vi "GetRoom.vi"(7 "Room Commands":T1, 8 "error in (no error)":errorcluster, 11 "Room Number":i32) -> (0 "error out":errorcluster, 2 "Flags JSON":string)   [LabVIEW 2015, in "RestApi.lvlib"]
uses:
  RestApi.lvlib
  TypeDef/GetRoomCommands.ctl
  TypeDef/FGVAction.ctl
  <vilib>/httpClient/LabVIEWHTTPClient.lvlib
panel:
  out "URL":string
  out "headers":string
  # "http://127.0.0.1:8001/WebService1/ReadFlag?Room={value}"
  # "http://127.0.0.1:8001/RivERWebService/"
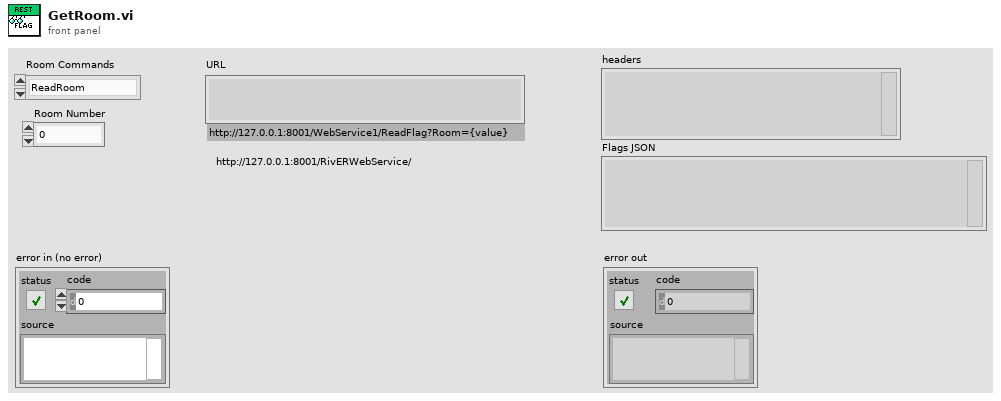
[diagram p1: front panel]
types:
  T1 = typedef "RestApi.lvlib/GetRoomCommands.ctl" = enum16{"ReadRoom", "ReadFlag", "ReadFlagState", "ReadFlagColor", "ReadBedVacant", "ReadPersonnel", "ReadRequests", "ReadBeaconID", "ReadBedURL"}
  T2 = typedef "FGVAction.ctl" = enum16{"Get", "Set"}
  T3 = typedef "LabVIEWHTTPClient.lvlib/ClientHandle.ctl" = refnum<k1>
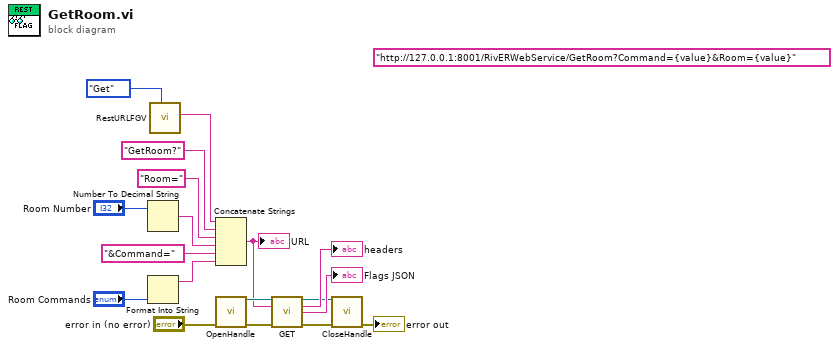
[diagram p0: block diagram]
diagram:
  (unwired) "http://127.0.0.1:8001/RivERWebService/GetRoom?Command={value}&Room={value}"
  n1 = Number To Decimal String(number="Room Number") -> (decimal integer string=w9:string)  [unwired: 1 in]
  n2 = Format Into String("Room Commands") -> (resulting string=w1:string)  [unwired: 3 in, 1 out]
  n3 = call "RestURLFGV.vi"("Action"=FGVAction."Get") -> ("URL"=w5:string)  [unwired: 9 in, 1 out]
  n4 = Concatenate Strings(w5, "GetRoom?" ("string"), "Room=" ("string"), w9, "&Command=" ("string"), w1) -> (w6:string)
  "URL" <- w6
  n5 = call <vilib>:"OpenHandle.vi"("error in (no error)"="error in (no error)") -> ("client handle out"=w18:T3, "error out"=w13:errorcluster)  [unwired: 13 in]
  n6 = call <vilib>:"GET.vi"("client handle"=w18, "url"=w6, "error in (no error)"=w13) -> ("client handle out"=w15:T3, "headers"=→"headers":string, "body"=→"Flags JSON":string, "error out"=w14:errorcluster)  [unwired: 9 in]
  n7 = call <vilib>:"CloseHandle.vi"("client handle"=w15, "error in (no error)"=w14) -> ("error out"=→"error out":errorcluster)  [unwired: 13 in]
